vi "PH_Sixpack_Switch.panel - defekt.vi"(0 "object ref":refnum<vi>, 5 "error in (no error)":errorcluster) -> (19 "error out":errorcluster)   [LabVIEW 2014, in "PH_Sixpack_Switch.lvlib"]
doc: "By this VI a hardware switch can be monitored and switched. \n\nThe indicators \"FALSE\", \"TRUE\" and \"SWITCH STATE\" show the value of the Beckhoff-Tag: blue indicates bad tag status reference problems, darkgreen false and lightgreen true. If everything is working fine, \"FALSE\" and \"SWITCH STATE\" should show the same value, while \"TRUE\" has the opposite value. The caption of the sensors for \"FALSE\" and \"TRUE\" are taken out of the database. In case of only one or no sensor these GUI elements are not shown at all.\n\nThe oval button switches. It should be in the same state as the \"SWITCH STATE\" indicator. \n\n\"Delete Instance\" disconnects and removes the instance from the PCS.\n\n\nLicense Agreement for this software:\n\nCopyright (C)\nGesellschaft für Schwerionenforschung, GSI\nPlanckstr. 1\n64291 Darmstadt\nGermany\n\nContact: D.Beck@gsi.de \n\nThis program is free software; you can redistribute it and/or modify it under the terms of the GNU General Public License as published by the Free Software Foundation; either version 2 of the license, or (at your option) any later version.\n\nThis program is distributed in the hope that it will be useful, but WITHOUT ANYW ARRANTY; without even the implied warranty of MERCHANTABILITY or FITNESS FOR A PARTICULAR PURPOSE. See the GNU General License for more details (http://www.gnu.org).\n\nGesellschaft für Schwerionenforschung, GSI\nPlanckstr. 1, 64291 Darmstadt, Germany\nFor all questions and ideas contact: M.Richter@gsi.de, H.Brand@gsi.de or D.Beck@gsi.de.\nLast update: 18-DEC-2002"
uses:
  PH_Sixpack_Switch.lvlib
  CSUser/DIMServiceTools/Status.ctl
  PH_Common/PH_Motion/PH_Motion.Axis Address.ctl
  PH_Common/PH_Motion/PH_Motion.Motor Type.ctl
  PH_Common/PH_Motion/PH_Motion.Axis Activity.ctl
  PH_Common/PH_Motion/PH_Motion.Endswitch Information.ctl
  PH_AxisGUI_BaseClass/PH_AxisGUI_BaseClass.Axis GUI Refs.ctl
  CSCore/CSObj/CSObj.lvlib
  CSCore/CSSystem/CSSystemLib/CSSystemLib.lvlib
  PH_PSDBWriter/PH_PSDBWriter.lvlib
  PH_AxisGUI_BaseClass/PH_AxisGUI_BaseClass.lvlib
panel:
  in  "Stop":bool caption="SetZero"
  out "PSDB Status":u32(colorbox)=6618880 caption="PSDB"
  in  "Tab Control":enum32{"Switch", "Switch Info", "Info"}(tab)=enum."Info"
  in  "Move":bool
  in  "Move in?":bool
  out "false-condition":T1 caption="Advanced"
  out "true-condition":T1 caption="Advanced"
  out "Endswitch Information":T2
  out "Axis Activity":T3
  out "Position":dbl
  out "Address":T4={"Instance"="N/A", "Motor Nr"=0}
  out "Switch Parameters":T6
  out "Status":T7 caption="Enabling State" items=["no info", "off/false/out", "on/true/in", "Failure", "Alarm", "Status 1", "Status 2", "Status 3"]
  in  "Exit":bool
  in  "Delete":bool
  out "loop counter":i32
  # "PCS"
  # "3.40"
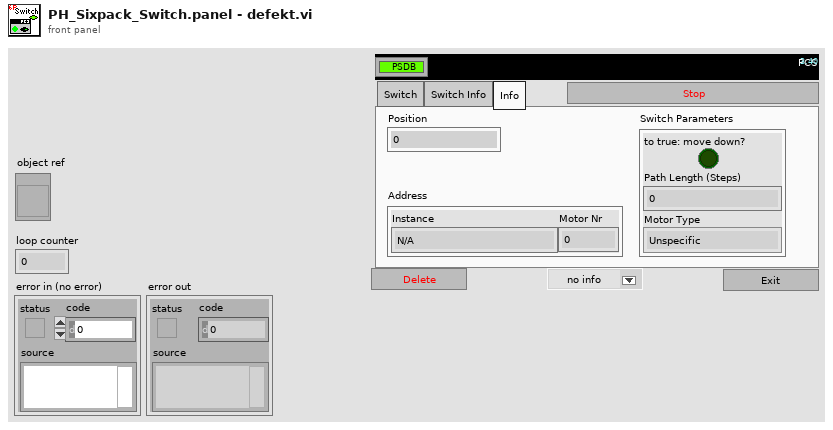
[diagram p1: front panel]
types:
  T1 = cluster{"AnalogIn":enum16{"<0.75V", "0.75...4V", ">4V", "99999"}, "ReferenceIn":bool}
  T2 = typedef "PH_Motion.Endswitch Information.ctl" = cluster{"Analog in / Endswitch 1":dbl, "Boolean in / Endswitch 2":bool}
  T3 = typedef "PH_Motion.Axis Activity.ctl" = enum16{"Inactive", "Ramp", "PI-Controller", "Rotation", "Reference Switch Search", "Reference SwitchSearch", "Mechanical Reference"}
  T4 = typedef "PH_Motion.Axis Address.ctl" = cluster{"Instance":string, "Motor Nr":i32}
  T5 = typedef "PH_Motion.Motor Type.ctl" = enum16{"Unspecific", "OWIS 49.120.2633", "OWIS 49.060.1033", "OWIS 43.040.2558", "Diamond Motion 2200 series", "OWIS 49.120.266B.MV6", "Calorimeter", "Linear Stage 1", "MICOS VT-80", "MICOS VT-80 S", "Standa Rotstage nt0.95A", "PUF RA 320.200", "PUF RA 800.200", "PUF RA 800.400", "PUF RA 400.50", "1324.nn.800.50", "1324.n9c.800.50"}
  T6 = cluster{"to true: move down?":bool, "Path Length (Steps)":dbl, "Motor Type":T5}
  T7 = typedef "Status.ctl" = i16
  T8 = typedef "PH_AxisGUI_BaseClass.lvlib/PH_AxisGUI_BaseClass.Axis GUI Refs.ctl" = cluster{"Back":refnum<vi>, "Forth":refnum<vi>, "Status":refnum<vi>, "Target":refnum<vi>, "Address":refnum<vi>, "Status Bar":refnum<vi>, "Settings":refnum<vi>, "Activity":refnum<vi>, "Endswitch":refnum<vi>}
  T9 = typedef "PH_Sixpack_Switch.lvlib/PH_Sixpack_Switch.i attribute.ctl" = cluster{"GUI Refs":cluster{"Delete":refnum<vi>, "Status":refnum<vi>, "Move":refnum<vi>, "Move in?":refnum<vi>, "Position":refnum<vi>, "true-condition":refnum<vi>, "false-condition":refnum<vi>, "Switch Parameters":refnum<vi>}, "Service ID Status":i32, "Status":T7, "remote controlled?":bool, "Switch Parameters":cluster{"to true: move down?":bool, "Path Length (Steps)":dbl, "Motor Type":T5}, "Info available":cluster{"motor type?":bool, "Scale linked?":bool, "Input linked?":bool, "Position linked?":bool}, "Move":bool, "Move in?":bool, "Position":dbl, "false-condition":cluster{"AnalogIn":enum16{"<0.75V", "0.75...4V", ">4V", "99999"}, "ReferenceIn":bool}, "true-condition":cluster{"AnalogIn":enum16{"<0.75V", "0.75...4V", ">4V", "99999"}, "ReferenceIn":bool}}
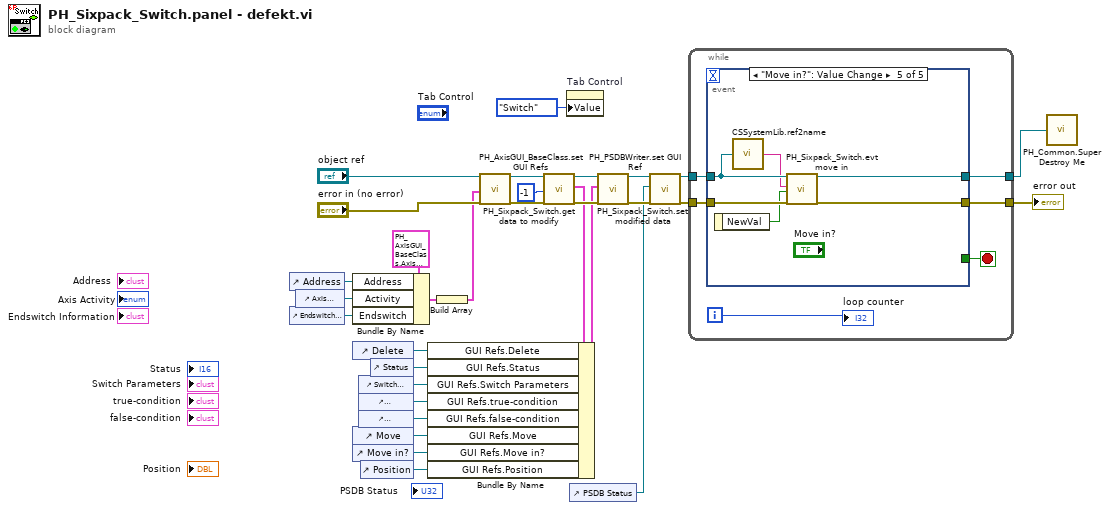
[diagram p0: block diagram]
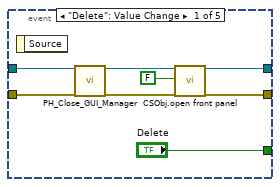
[diagram p2: hidden frame]
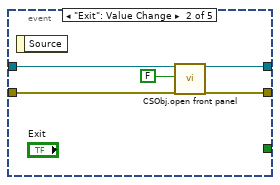
[diagram p3: hidden frame]
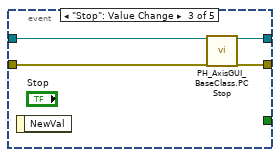
[diagram p4: hidden frame]
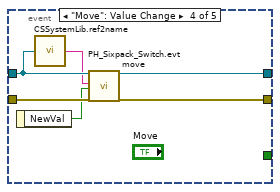
[diagram p5: hidden frame]
diagram:
  n1 = control-ref of="Address"() -> (w2:refnum<vi>)
  n2 = control-ref of="Endswitch Information"() -> (w4:refnum<vi>)
  n3 = control-ref of="Axis Activity"() -> (w3:refnum<vi>)
  n4 = Bundle By Name(cluster=T8 {"Back"=refnum, "Forth"=refnum, "Status"=refnum, "Target"=refnum, "Address"=refnum, "Status Bar"=refnum, "Settings"=refnum, "Activity"=refnum, "Endswitch"=refnum} ("GUI Refs"), "Address"=w2, "Activity"=w3, "Endswitch"=w4) -> (w6:T8)
  n5 = control-ref of="Delete"() -> (w26:refnum<vi>)
  n6 = control-ref of="Move"() -> (w21:refnum<vi>)
  n7 = control-ref of="Move in?"() -> (w20:refnum<vi>)
  n8 = control-ref of="Switch Parameters"() -> (w11:refnum<vi>)
  n9 = control-ref of="true-condition"() -> (w18:refnum<vi>)
  n10 = control-ref of="false-condition"() -> (w17:refnum<vi>)
  n11 = control-ref of="Position"() -> (w19:refnum<vi>)
  n12 = control-ref of="Status"() -> (w24:refnum<vi>)
  n13 = Build Array(w6) -> (w5:T8[])
  n14 = call "PH_AxisGUI_BaseClass.set GUI Refs.vi"("i ref in"="object ref", "Axis GUI Refs"=w5, "error in"="error in (no error)") -> ("i ref out"=w8:refnum<vi>, "error out"=w10:errorcluster)  [unwired: 15 in]
  n15 = call "PH_Sixpack_Switch.get data to modify.vi"("i ref in"=w8, "ms timeout (10000)"=-1, "error in (no error)"=w10) -> ("i ref out"=w31:refnum<vi>, "i attribute"=w29:T9, "error out"=w30:errorcluster)  [unwired: 13 in, 1 out]
  n16 = Bundle By Name(cluster=w29, "GUI Refs.Delete"=w26, "GUI Refs.Status"=w24, "GUI Refs.Switch Parameters"=w11, "GUI Refs.true-condition"=w18, "GUI Refs.false-condition"=w17, "GUI Refs.Move"=w21, "GUI Refs.Move in?"=w20, "GUI Refs.Position"=w19) -> (w28:T9)
  n17 = property on="Tab Control" class="TabCtl (strict)"("Value"=enum32{"Switch", "Switch Info", "Info"}."Switch" ("Tab Control")) -> ()  [unwired: 2 in, 2 out]
  n18 = control-ref of="PSDB Status"() -> (w12:refnum<vi>)
  n19 = call "PH_Sixpack_Switch.set modified data.vi"("i ref in"=w31, "i attribute"=w28, "error in (no error)"=w30) -> ("i ref out"=w14:refnum<vi>, "error out"=w16:errorcluster)  [unwired: 15 in]
  n20 = call "PH_PSDBWriter.set GUI Ref.vi"("i ref in"=w14, "Ref PSDB Status"=w12, "error in"=w16) -> ("i ref out"=w13:refnum<vi>, "error out"=w15:errorcluster)  [unwired: 15 in]
  n21 = while {
    tunnel: w13 -> [w33]
    tunnel: [w32] -> w23
    tunnel: w15 -> [w35]
    tunnel: [w34] -> w22
    i -> [w36]
    stop <- w37 stop-if-true
    n22 = event shown="[4] \"Move in?\": Value Change" {
      selector: _ -> [_ _ _ _ _]
      dyn-events: _ -> [_ _ _ _ _]
      timeout: _ -> [_ _ _ _ _]
      tunnel: ["Delete" _ _ _ _] -> w37
      tunnel: w33 -> [w41 w49 w52 w57 w63]
      tunnel: w35 -> [w39 w48 w51 w60 w66]
      tunnel: [w43 w47 w53 w58 w64] -> w34
      tunnel: [w42 w46 w54 w59 w65] -> w32
      event "Delete": Value Change {
        n23 = event-data() -> ()  [unwired: 1 in, 1 out]
        n24 = call "PH_Close_GUI_Manager.vi"("i ref in"=w41, "error in"=w39) -> ("i ref out"=w40:refnum<vi>, "error out"=w38:errorcluster)  [unwired: 16 in]
        n25 = call "CSObj.open front panel.vi"("i ref in"=w40, "frontPanelOpen"=FALSE ("front panel open"), "error in (no error)"=w38) -> ("i ref out"=w42:refnum<vi>, "error out"=w43:errorcluster)  [unwired: 15 in]
      }
      event "Exit": Value Change {
        n26 = event-data() -> ()  [unwired: 1 in, 1 out]
        n27 = call "CSObj.open front panel.vi"("i ref in"=w49, "frontPanelOpen"=FALSE ("front panel open"), "error in (no error)"=w48) -> ("i ref out"=w46:refnum<vi>, "error out"=w47:errorcluster)  [unwired: 15 in]
      }
      event "Stop": Value Change {
        n28 = event-data() -> ()  [unwired: 1 in, 1 out]
        n29 = call "PH_AxisGUI_BaseClass.PC Stop.vi"("VI in"=w52, "error in (no error)"=w51) -> ("VI out"=w54:refnum<vi>, "error out"=w53:errorcluster)  [unwired: 16 in]
      }
      event "Move": Value Change {
        n30 = event-data() -> ("NewVal"=w55:bool)  [unwired: 1 in]
        n31 = call "CSSystemLib.ref2name.vi"("obj refnum"=w57) -> ("name"=w56:string)
        n32 = call "PH_Sixpack_Switch.evt move.vi"("i ref in"=w57, "Instance"=w56, "Move"=w55, "error in (no error)"=w60) -> ("i ref out"=w59:refnum<vi>, "error out"=w58:errorcluster)  [unwired: 14 in]
      }
      event "Move in?": Value Change {
        n33 = event-data() -> ("NewVal"=w61:bool)  [unwired: 1 in]
        n34 = call "CSSystemLib.ref2name.vi"("obj refnum"=w63) -> ("name"=w62:string)
        n35 = call "PH_Sixpack_Switch.evt move in.vi"("i ref in"=w63, "Instance"=w62, "Move In?"=w61, "error in (no error)"=w66) -> ("i ref out"=w65:refnum<vi>, "error out"=w64:errorcluster)  [unwired: 14 in]
      }
    }
    "loop counter" <- w36
  }
  "error out" <- w22
  n36 = call "PH_Common.Super Destroy Me.vi"("i ref out"=w23) -> ()
